vi "NI 9470 Duty Cycle (Host).vi"() -> ()   [LabVIEW 2023]
uses:
  <vilib>/userDefined/High Color/nirio_resource_hc.ctl
  <vilib>/LabVIEW Targets/FPGA/cRIO/shared/nicrio_ModuleControls/nicrio_cRIO-9470_DataRatesRing.ctl
  <vilib>/FPGAPlugInAG/cRIO-9049/niLvFpga_Open_cRIO-9049.vi
  <vilib>/rvi/interface/common/dynamic/niFpgaDynamicAddResources.vi
  <vilib>/FPGAPlugInAG/Dynamic/niLvFpga_Reset_Dynamic.vi
  <vilib>/FPGAPlugInAG/Dynamic/niLvFpga_Run_Dynamic.vi
  <vilib>/Utility/error.llb/Error Cluster From Error Code.vi
  <vilib>/rvi/errors/niLvFpgaAdjustHostInterfaceError.vi
  <vilib>/FPGAPlugInAG/Dynamic/niLvFpga_Close_Dynamic.vi
  <vilib>/rvi/interface/nirviOpenFPGA/nirviOpenFPGA.xnode
  Projects/FPGA Bitfiles/grimmrio_FPGATarget_9470ExampleFPGAC_fUC4GTl-uk0.lvbitx
  <vilib>/rvi/interface/nirviMethod/nirviMethod.xnode
  <vilib>/rvi/interface/nirviReadWriteControl/nirviReadWriteControl.xnode
  <vilib>/rvi/interface/nirviCloseFPGA/nirviCloseFPGA.xnode
  <vilib>/rvi/interface/Simulation/niFpgaSimulationCallBeginRW.vi
  <vilib>/FPGAPlugInAG/Dynamic/niLvFpga_ReadFifo_Dynamic.vi
  <vilib>/rvi/errors/niLvFpgaMergeErrorWithErrorCode.vi
  NiFpgaLv.dll
panel:
  out "Waveform Chart":dbl[](graph)
  out "FIFO Timeout":bool
  out "FPGA Error Out":errorcluster
  out "Host Error Out":errorcluster
  out "Waveform Graph":waveform(dbl)[](graph)
  in  "Dither Divisor":u16
  in  "Dither Amplitude":fxp<+,17,7>
  out "Module Temperature":fxp<+/-,12,9>
  in  "Data Rate":T1 items=["3.200 kS/s (NI 9470)", "3.125 kS/s (NI 9470)", "2.560 kS/s (NI 9470)", "2.000 kS/s (NI 9470)"]
  in  "PWM Divisor":u16
  in  "CH1 Enable on Fault":bool
  out "Voltage (V)":fxp<+,12,6>[](array[numeric])
  out "CH1 Overcurrent":bool
  out "CH1 Pwr Fault":bool
  in  "Duty Cycle %":fxp<+,17,7>[](array[numeric])=[0.0, 0.0, 0.0, 0.0, 0.0, 0.0, 0.0, 0.0]
  in  "Elements to Read":u32=5000
  out "PWM Period (s)":dbl
  in  "RIO Device":T2="RIO0"
  in  "Stop":bool
  in  "CH0 Enable on Fault":bool
  out "CH0 Overcurrent":bool
  out "CH0 Pwr Fault":bool
  out "Module Overtemp":bool
  # "Overview: Demonstrates how to set a Duty Cycle % output and readback Average Current with the NI 9470\nRequirements: LabVIEW Full Development System, LV FPGA, and NI RIO\nInstructions: \n1. Run the VI."
  # "Measurement Parameters and Setpoint"
  # "Module Readback and Fault Status"
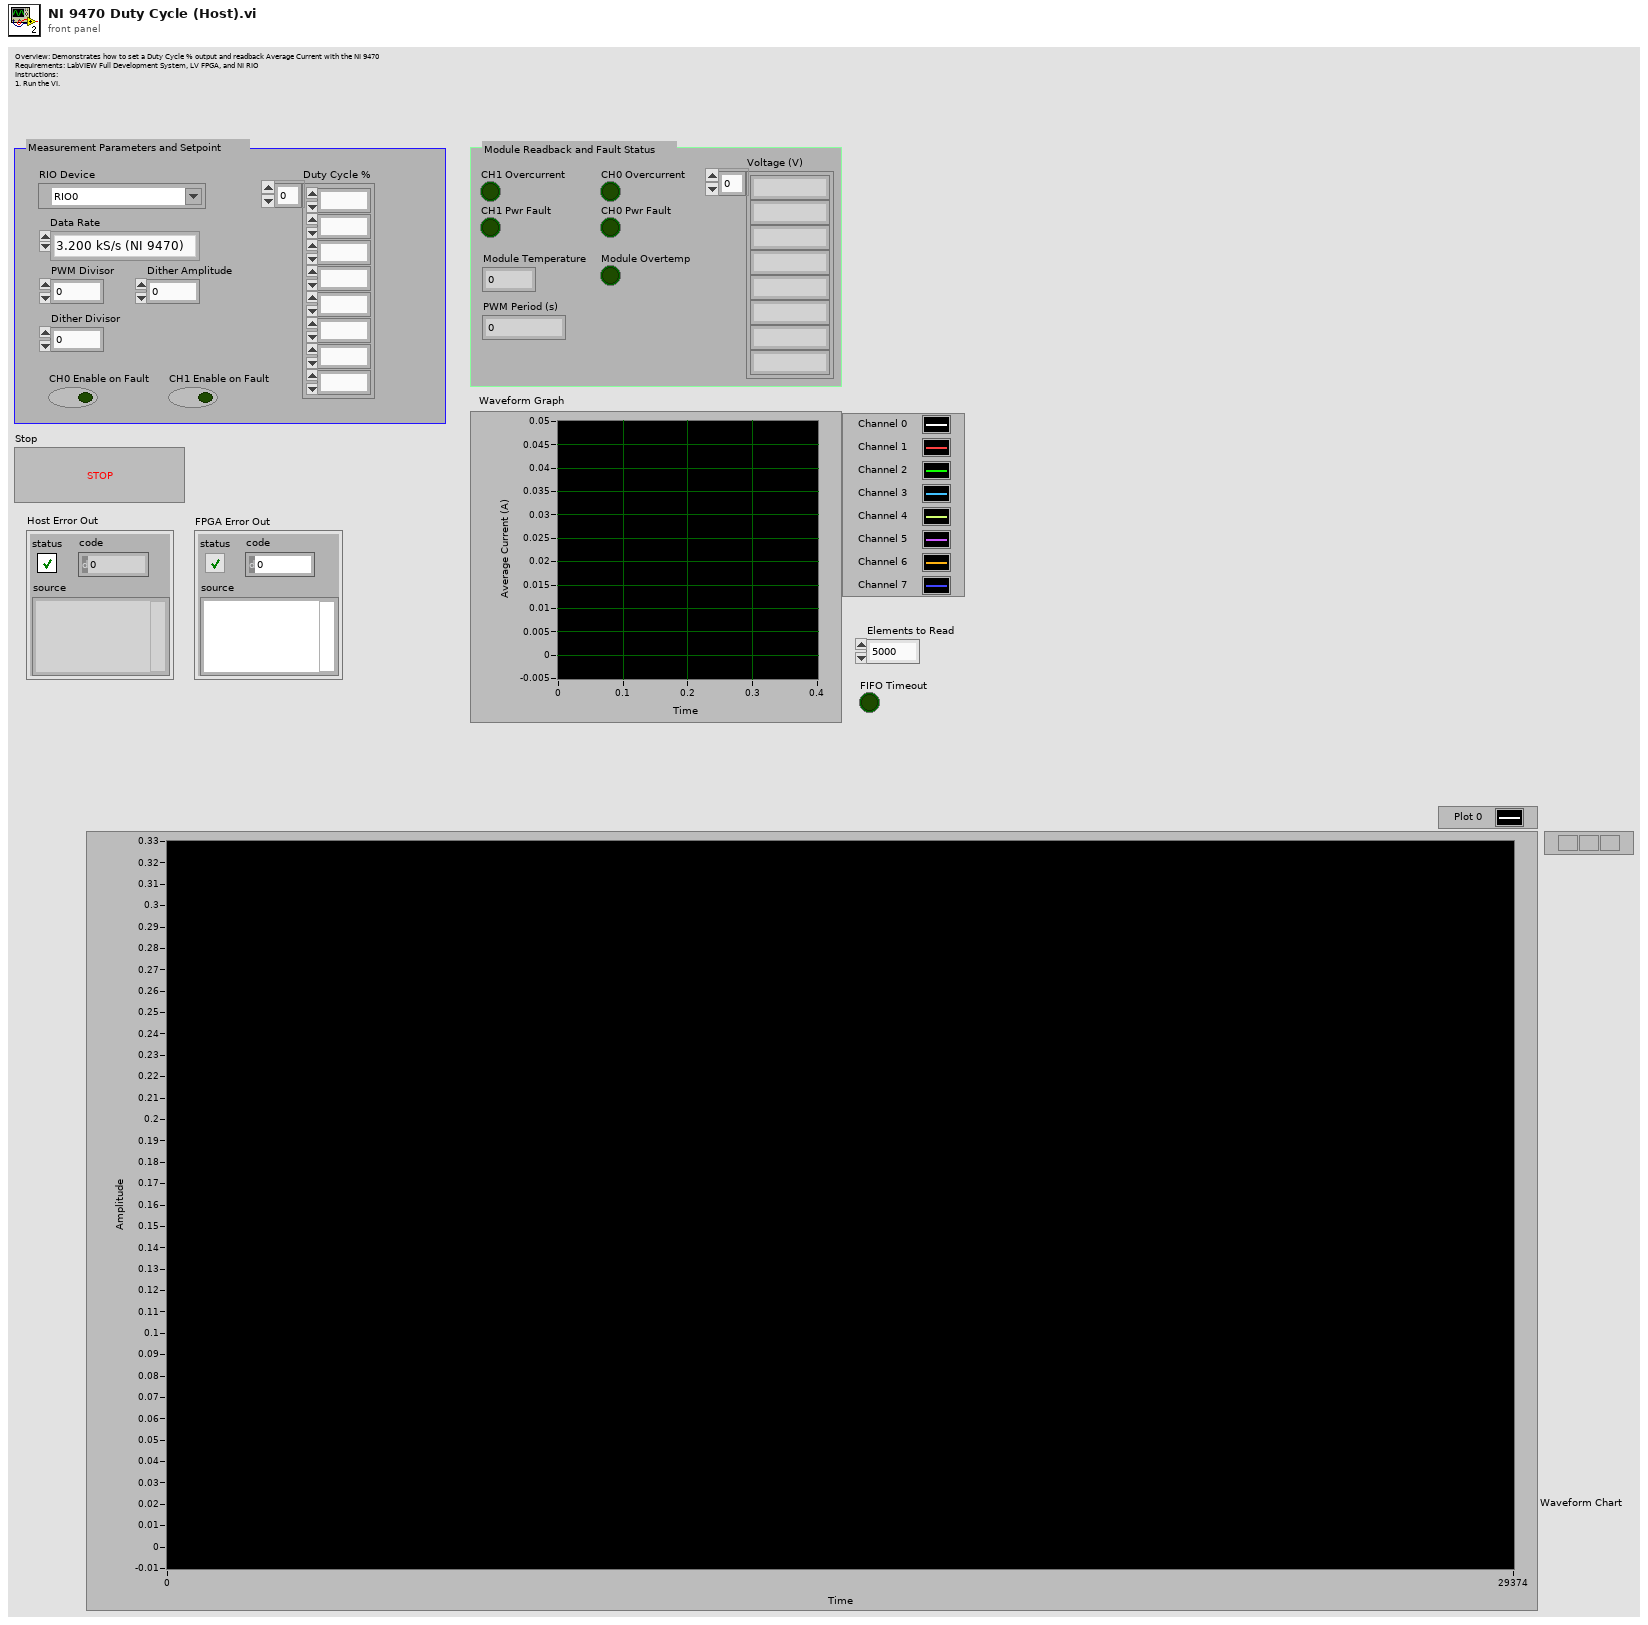
[diagram p1: front panel]
types:
  T1 = typedef "nicrio_cRIO-9470_DataRatesRing.ctl" = u8
  T2 = typedef "nirio_resource_hc.ctl" = tag
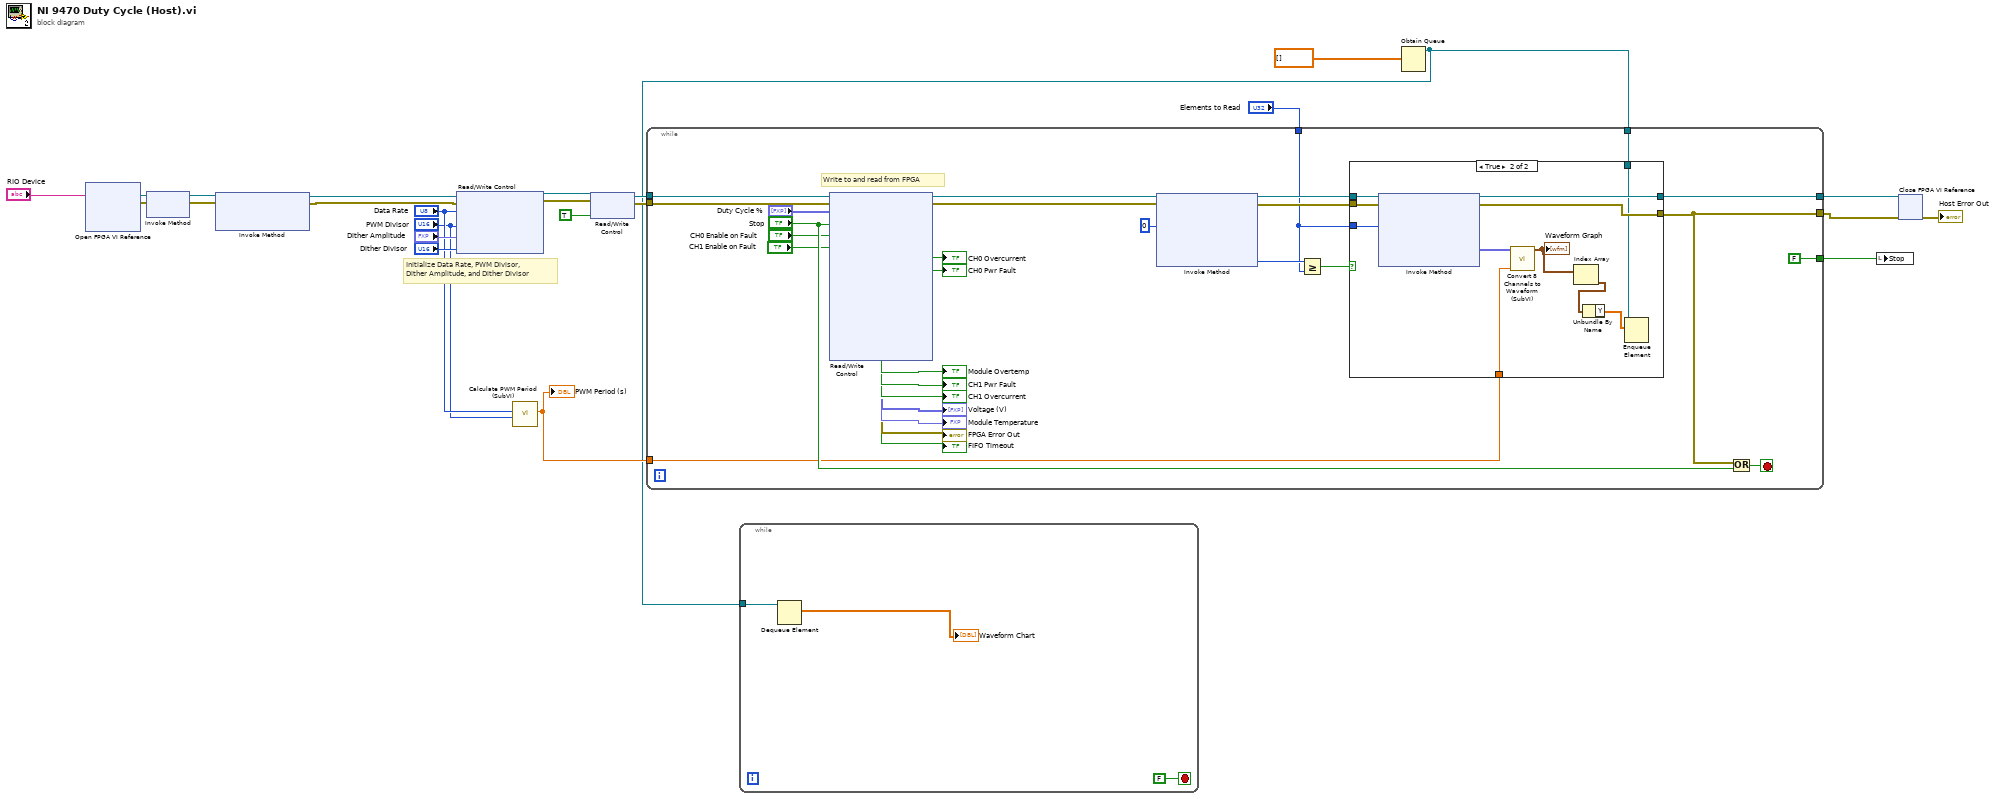
[diagram p0: block diagram]
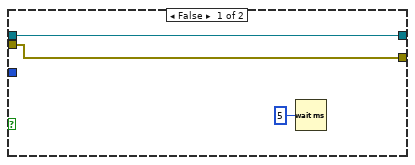
[diagram p2: hidden frame]
diagram:
  # "Initialize Data Rate, PWM Divisor, \nDither Amplitude, and Dither Divisor"
  n1 = xnode "Open FPGA VI Reference"("resource name"="RIO Device") -> ("FPGA VI Reference Out"=w18:refnum<k20>, "error out"=w17:errorcluster)  [unwired: 1 in]
  n2 = xnode "Invoke Method"("FPGA VI Reference In"=w18, "error in"=w17) -> ("FPGA VI Reference Out"=w24:refnum<k20>, "error out"=w23:errorcluster)
  n3 = xnode "Invoke Method"("FPGA VI Reference In"=w24, "error in"=w23) -> ("FPGA VI Reference Out"=w12:refnum<k20>, "error out"=w11:errorcluster)  [unwired: 1 in]
  n4 = xnode "Read/Write Control"("FPGA VI Reference In"=w12, "error in"=w11, "Data Rate"="Data Rate", "PWM Divisor"="PWM Divisor", "Dither Amplitude"="Dither Amplitude", "Dither Divisor"="Dither Divisor") -> ("FPGA VI Reference Out"=w14:refnum<k20>, "error out"=w13:errorcluster)
  n5 = call "Calculate PWM Period (SubVI).vi"("PWM Divisor"="PWM Divisor", "Data Rate"="Data Rate") -> ("PWM Period"=w3:dbl)  [unwired: 9 in]
  "PWM Period (s)" <- w3
  n6 = xnode "Read/Write Control"("FPGA VI Reference In"=w14, "error in"=w13, "Ready?"=TRUE) -> ("FPGA VI Reference Out"=w16:refnum<k20>, "error out"=w15:errorcluster)
  n7 = Obtain Queue(element data type=dbl[] [] ("Y")) -> (queue out=w1:refnum<queue>)  [unwired: 4 in, 2 out]
  n8 = while {
    tunnel: [w41] -> w20
    tunnel: w16 -> [w49]
    tunnel: w15 -> [w48]
    tunnel: [FALSE] -> w21
    tunnel: [w47] -> w10
    tunnel: "Elements to Read" -> [w27]
    tunnel: w3 -> [w26]
    tunnel: w1 -> [w25]
    stop <- w42 stop-if-true
    # "Write to and read from FPGA"
    n9 = xnode "Read/Write Control"("FPGA VI Reference In"=w49, "error in"=w48, "Duty Cycle %"="Duty Cycle %", "stop"="Stop", "CH0 Enable on Fault"="CH0 Enable on Fault", "CH1 Enable on Fault"="CH1 Enable on Fault") -> ("FPGA VI Reference Out"=w34:refnum<k20>, "error out"=w33:errorcluster, "CH0 Overcurrent"=→"CH0 Overcurrent":bool, "CH0 Pwr Fault"=→"CH0 Pwr Fault":bool, "Module Overtemp"=→"Module Overtemp":bool, "CH1 Pwr Fault"=→"CH1 Pwr Fault":bool, "CH1 Overcurrent"=→"CH1 Overcurrent":bool, "Voltage (V)"=→"Voltage (V)":fxp<+,12,6>[], "Module Temperature"=→"Module Temperature":fxp<+/-,12,9>, "error out"=→"FPGA Error Out":errorcluster, "FIFO Timeout"=→"FIFO Timeout":bool)
    n10 = xnode "Invoke Method"("FPGA VI Reference In"=w34, "error in"=w33, "Number of Elements"=u32 0) -> ("FPGA VI Reference Out"=w32:refnum<k20>, "error out"=w31:errorcluster, "Elements Remaining"=w29:u32)  [unwired: 1 in, 1 out]
    n11 = Greater Or Equal?(x=w29, y=w27) -> (x >= y?=w28:bool)
    n12 = case shown="True" w28 {
      tunnel: [w55 w67] -> w47
      tunnel: [w54 w65] -> w41
      tunnel: w32 -> [w55 w64]
      tunnel: w31 -> [w54 w63]
      tunnel: w27 -> [_ w62]
      tunnel: w26 -> [_ w61]
      tunnel: w25 -> [_ w57]
      frame False {
        n13 = Wait (ms)(milliseconds to wait=u32 5) -> ()  [unwired: 1 out]
      }
      frame True {
        n14 = xnode "Invoke Method"("FPGA VI Reference In"=w64, "error in"=w63, "Number of Elements"=w62) -> ("FPGA VI Reference Out"=w67:refnum<k20>, "error out"=w65:errorcluster, "Data"=w66:fxp<+/-,16,3>[])  [unwired: 1 in, 1 out]
        n15 = call "Convert 8 Channels to Waveform (SubVI).vi"("dt"=w61, "Data"=w66) -> ("appended array"=w60:waveform(dbl)[])  [unwired: 9 in]
        "Waveform Graph" <- w60
        n16 = Index Array(array=w60) -> (element=w59:waveform(dbl))  [unwired: 1 in]
        n17 = Unbundle By Name(w59) -> ("Y"=w58:dbl[])
        n18 = Enqueue Element(queue=w57, element=w58) -> ()  [unwired: 2 in, 3 out]
      }
    }
    n19 = Or(x=w41, y="Stop") -> (x .or. y?=w42:bool)
  }
  n20 = while {
    tunnel: w1 -> [w70]
    stop <- FALSE stop-if-true
    n21 = Dequeue Element(queue=w70) -> (element=→"Waveform Chart":dbl[])  [unwired: 2 in, 3 out]
  }
  n22 = local write "Stop"(w21) -> ()
  n23 = xnode "Close FPGA VI Reference"("FPGA VI Reference In"=w10, "error in"=w20) -> ("error out"=→"Host Error Out":errorcluster)
